vi "Load System Settings From ini File.vi"(8 "error in":errorcluster) -> (0 "error out":errorcluster, 2 "INI error":bool)   [LabVIEW 2013]
doc: "Loads all System Settings from an INI file."
uses:
  INI Section Enum.ctl
  Image Acquisition/Image Acquisition Settings FG Enum.ctl
  Debug/Debug Settings FG Enum.ctl
  Image Processing/Mask ROI FG Enum.ctl
  Common/File IO/INI/Read write mode.ctl
  Globals/Simulation Settings Global.vi
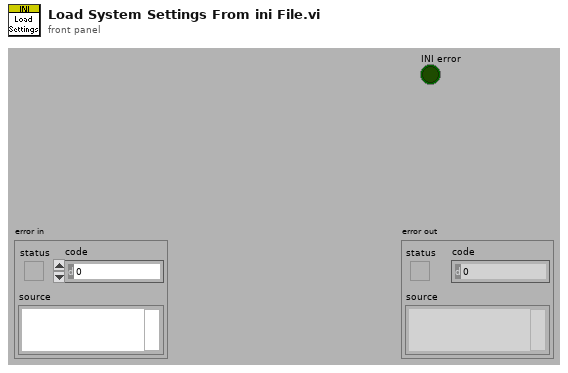
[diagram p1: front panel]
types:
  T1 = typedef "Image Acquisition Settings FG Enum.ctl" = enum16{"Read", "Write"}
  T2 = typedef "Debug Settings FG Enum.ctl" = enum16{"Read", "Write"}
  T3 = typedef "Mask ROI FG Enum.ctl" = enum16{"Read", "Write", "Enable Background", "Disable Background"}
  T4 = typedef "Read write mode.ctl" = enum16{"Read", "Write"}
  T5 = typedef "INI Section Enum.ctl" = enum16{"Simulation", "Image Attributes", "ROI", "Debug"}
  T6 = typedef "Simulation Settings Cluster.ctl" = cluster{"Sim Enabled?":bool, "Sim Path":path}
  T7 = typedef "Acquisition Settings Cluster.ctl" = cluster{"Image Width":u32, "Image Height":u32, "Frames To Acquire":u32, "Signal Mapping":enum8{"Standard", "Basler 10-tap", "Vosskühler 10-tap"}, "DMA Buffer Size\n(In Images)":u32}
  T8 = typedef "Debug Settings Cluster.ctl" = cluster{"Save Images?":bool, "Save Image Path":path}
  T9 = typedef "Mask ROI Cluster.ctl" = cluster{"left annulus":T10, "right annulus":T10, "Threshold Range":cluster{"Lower value":dbl, "Upper value":dbl}, "[Avg BG]":u8[], "Number of Sectors":u8, "Left ROI":T11, "Right ROI":T11, "Left Start Angle Duty Cycle":fxp<+,8,0>, "Left End Angle Duty Cycle":fxp<+,8,0>, "Right End Angle Duty Cycle":fxp<+,8,0>, "Right Start Angle Duty Cycle":fxp<+,8,0>, "[Sector ROIs]":T11[], "Consecutive Sector Threshold":u8}
  T10 = typedef "IMAQ Circle" = cluster{"Center X":i32, "Center Y":i32, "Inner Radius":i32, "Outer Radius":i32, "Start Angle":dbl, "End Angle":dbl}
  T11 = typedef "ROI Descriptor" = cluster{"Global Rectangle":i32[], "Contours":cluster{"ID":enum32{"External", "Internal"}, "Type":u32, "Coordinates":i32[]}[]}
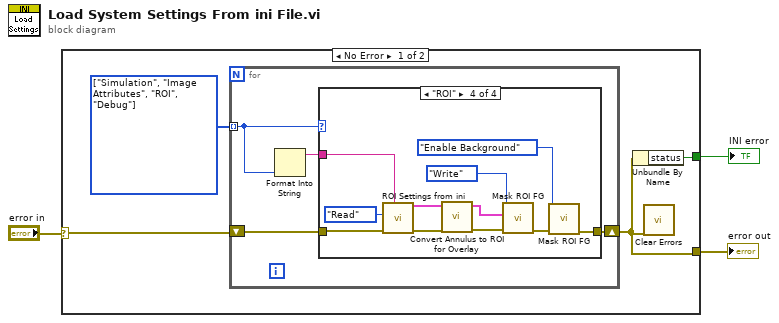
[diagram p0: block diagram]
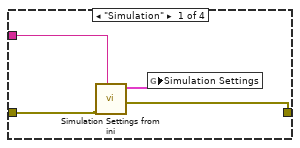
[diagram p2: hidden frame]
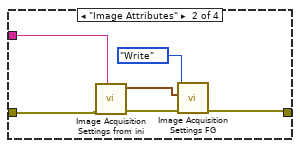
[diagram p3: hidden frame]
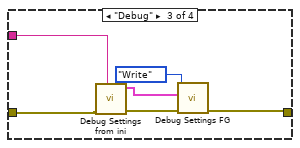
[diagram p4: hidden frame]
diagram:
  n1 = case shown="No Error" "error in" {
    selector: "error in" -> [w5 w39]
    tunnel: [w6 FALSE ("status")] -> w3
    tunnel: [w4 w39] -> w1
    frame No Error {
      w7 = T5[] [enum."Simulation", enum."Image Attributes", enum."ROI", enum."Debug"] items=["Simulation", "Image Attributes", "ROI", "Debug"]
      n2 = for {
        shift-right: [w10] -> w4
        shift-left: w5 -> [w11]
        tunnel: w7 -> [w9] mode=indexing
        n3 = Format Into String(w9) -> (resulting string=w8:string)  [unwired: 3 in, 1 out]
        n4 = case shown="\"ROI\"" w9 {
          tunnel: w11 -> [w15 w21 w27 w38]
          tunnel: [w13 w18 w24 w29] -> w10
          tunnel: w8 -> [w14 w20 w26 w37]
          frame "Simulation" {
            n5 = call "Simulation Settings from ini.vi"("Section"=w14, "error in (no error)"=w15) -> ("error out"=w13:errorcluster, "Simulation Settings Out"=w12:T6)  [unwired: 7 in, 1 out]
            n6 = global write "Simulation Settings Global.vi" "Simulation Settings"(w12) -> ()
          }
          frame "Image Attributes" {
            n7 = call "Image Acquisition Settings from ini.vi"("Section"=w20, "error in (no error)"=w21) -> ("error out"=w19:errorcluster, "Acquisition Settings Cluster"=w16:T7)  [unwired: 7 in, 1 out]
            n8 = call "Image Acquisition Settings FG.vi"("error in (no error)"=w19, "Acquisition Settings In"=w16, "Operation"=Image_Acquisition_Settings_FG_Enum."Write") -> ("error out"=w18:errorcluster)  [unwired: 7 in, 1 out]
          }
          frame "Debug" {
            n9 = call "Debug Settings from ini.vi"("Section"=w26, "error in (no error)"=w27) -> ("error out"=w25:errorcluster, "Debug Settings Cluster"=w23:T8)  [unwired: 7 in, 1 out]
            n10 = call "Debug Settings FG.vi"("error in (no error)"=w25, "Debug Settings In"=w23, "Operation"=Debug_Settings_FG_Enum."Write") -> ("error out"=w24:errorcluster)  [unwired: 7 in, 1 out]
          }
          frame "ROI" {
            n11 = call "ROI Settings from ini.vi"("Section"=w37, "error in (no error)"=w38, "Operation"=Read_write_mode."Read") -> ("error out"=w34:errorcluster, "Mask ROI Out"=w32:T9)  [unwired: 6 in, 1 out]
            n12 = call "Convert Annulus to ROI for Overlay.vi"("error in (no error)"=w34, "Mask ROI In"=w32) -> ("error out"=w33:errorcluster, "Mask ROI Out"=w31:T9)  [unwired: 8 in]
            n13 = call "Mask ROI FG.vi"("error in (no error)"=w33, "Mask ROI In"=w31, "Operation"=Mask_ROI_FG_Enum."Write") -> ("error out"=w30:errorcluster)  [unwired: 7 in, 1 out]
            n14 = call "Mask ROI FG.vi"("error in (no error)"=w30, "Operation"=Mask_ROI_FG_Enum."Enable Background") -> ("error out"=w29:errorcluster)  [unwired: 8 in, 1 out]
          }
        }
      }
      n15 = Unbundle By Name(w4) -> ("status"=w6:bool)
      n16 = call <vilib>:"Clear Errors.vi"("error in (no error)"=w4) -> ()  [unwired: 7 out]
    }
    frame Error {
      (unwired) TRUE ("INI Updated")
    }
  }
  "error out" <- w1
  "INI error" <- w3
